vi "backemfconstant.vi"(4 "Cutoff Frequency":i32=10000, 6 "Noise Band":dbl=0.01, 7 "rate":i32=100000, 8 "Pole Pair":i32=5, 9 "Back  EMF data":dbl[](array[numeric])) -> (0 "Variance":dbl=3.1792063558717476e-05, 1 "ZCP":i32[](array[numeric]), 2 "Filiter Voltage":dbl[](array[numeric]), 3 "Mean":dbl=0.07460512010090932, 5 "B-EMF":dbl[](graph)=[0.07481589133166745, 0.07511337105786742, 0.0741529055838003, 0.07537265906376046, 0.07508825632115766, 0.07557435638030187, 0.0743975577603694, 0.07492228255252237, 0.07463056189525759, 0.0758438201846894, 0.07482290613743812, 0.07511679185821236, 0.07415273237871953, 0.07537876454285714, 0.07509791250440986, 0.07558596112071256, 0.0743927080181082, 0.07491881845090724, 0.07463770660483883, 0.07585304335523971, 0.07481316335164553, 0.07513961162760209, 0.07414004510655407, 0.0753934869747215, 0.07509271635198714, 0.07559592041285612, 0.07439296782572931, 0.07493276145990817, 0.07463588795149087, 0.07587720546400528, 0.07480203492520691, 0.07514974412482635, 0.07413324680713437, 0.07542358135750299, 0.07508440250811083, 0.07560570649991886, 0.07438603962249907, 0.07495536472294693, 0.07461891385357669, 0.07588144898848384, 0.07480381027728465, 0.07516195508301972, 0.07413138485251623, 0.07541942443556485, 0.07507565565153261, 0.07562294040545418, 0.07437421837573739, 0.07496484770111837, 0.07462229135265147, 0.07589993863085463, 0.07480216482901747, 0.07518568417908342, 0.07412164206672368, 0.07543691814872129, 0.07506110642474902, 0.07564398482276614, 0.07437668654813819, 0.07498160529268162, 0.07461267847066942, 0.0759097247179174, 0.07477362929196277, 0.07519404132422994, 0.07411445405587225, 0.07546108025748688, 0.07506634587844192, 0.07565281828188475, 0.07436131459722098, 0.07499658753216708, 0.07460471103695462, 0.07593150525682257, 0.0747739324008541, 0.07521118862722488, 0.07411661911938174, 0.075469350800093, 0.07505032440847191, 0.07567741340335221, 0.07435451629780128, 0.07502092284601342, 0.07459782613499454, 0.0759478731369541, 0.07476483913411439, 0.07523058759626963, 0.07409336633729012, 0.07548000291255955, 0.07504733662082885, 0.07569139971362333, 0.07435061918348428, 0.0750335235156385, 0.0745818912675649, 0.07596948047077853, 0.07476141833376944, 0.07525267124406612, 0.07408821348613759, 0.07550827864199311, 0.07503378332325962, 0.07571058217631717, 0.07433632976432183, 0.07505898466250974, 0.0745710659500176, 0.07598351008231984, 0.07475838724485617, 0.07526722047084973, 0.07407912021939786, 0.07552399700307182, 0.07501602980248206, 0.07573383495840878, 0.0743232094794545, 0.07508344988016666, 0.07455508778131775, 0.07600464110217219, 0.07473353231576757, 0.07529501988631122, 0.07406253583291537, 0.0755460806508683, 0.07500832217638835, 0.07575197819061805, 0.07430298778627613, 0.07510068378570196, 0.0745526629101872, 0.07604226990596659, 0.0747173376407168, 0.07531303321470993, 0.07405010836837107, 0.07557439968157206, 0.074991304777204, 0.07578306850261392, 0.07429489044875075, 0.0751250624008185, 0.07452858740396197, 0.07605456746670036, 0.07470581950284645, 0.0753423914758982, 0.07402646587484775, 0.07559358214426588, 0.07497147279545732, 0.07580671099613724, 0.07426800035996324, 0.07516173857666877, 0.07450693676886735, 0.07607426954463645, 0.07468577101474887, 0.07537097031422309, 0.07399957578606026, 0.07563593078651094, 0.07496328885539158, 0.0758321721430085, 0.07424877459599921, 0.07519157315182916, 0.07447896414832511, 0.07611419331575092, 0.07466234502757649, 0.07539301066074941, 0.07397181967186896, 0.07566411991340413, 0.07492154643092916, 0.07586607703756665, 0.0742194596360811, 0.07522162423334047, 0.07445055851508102, 0.07615680176561711, 0.07463056189525759, 0.07543172199629856, 0.07394415016021806, 0.07570560253024541, 0.0748928376887937, 0.07590998452553853, 0.07418278346023084, 0.07526743697720066, 0.07441184717953182, 0.07620157527899274, 0.07459211036732954, 0.0754861949941966, 0.07390513571577755, 0.075761114758628, 0.07485213449481584, 0.07596172954341465, 0.07414134414465974, 0.07530259760859431, 0.0])   [LabVIEW 2013]
uses:
  <vilib>/Analysis/NI_AALBase.lvlib
panel:
  out "standard deviation":dbl format="%0.5f"
  out "B-EMF 2":dbl[](graph)=[0.07481589133166745, 0.07511337105786742, 0.0741529055838003, 0.07537265906376046, 0.07508825632115766, 0.07557435638030187, 0.0743975577603694, 0.07492228255252237, 0.07463056189525759, 0.0758438201846894, 0.07482290613743812, 0.07511679185821236, 0.07415273237871953, 0.07537876454285714, 0.07509791250440986, 0.07558596112071256, 0.0743927080181082, 0.07491881845090724, 0.07463770660483883, 0.07585304335523971, 0.07481316335164553, 0.07513961162760209, 0.07414004510655407, 0.0753934869747215, 0.07509271635198714, 0.07559592041285612, 0.07439296782572931, 0.07493276145990817, 0.07463588795149087, 0.07587720546400528, 0.07480203492520691, 0.07514974412482635, 0.07413324680713437, 0.07542358135750299, 0.07508440250811083, 0.07560570649991886, 0.07438603962249907, 0.07495536472294693, 0.07461891385357669, 0.07588144898848384, 0.07480381027728465, 0.07516195508301972, 0.07413138485251623, 0.07541942443556485, 0.07507565565153261, 0.07562294040545418, 0.07437421837573739, 0.07496484770111837, 0.07462229135265147, 0.07589993863085463, 0.07480216482901747, 0.07518568417908342, 0.07412164206672368, 0.07543691814872129, 0.07506110642474902, 0.07564398482276614, 0.07437668654813819, 0.07498160529268162, 0.07461267847066942, 0.0759097247179174, 0.07477362929196277, 0.07519404132422994, 0.07411445405587225, 0.07546108025748688, 0.07506634587844192, 0.07565281828188475, 0.07436131459722098, 0.07499658753216708, 0.07460471103695462, 0.07593150525682257, 0.0747739324008541, 0.07521118862722488, 0.07411661911938174, 0.075469350800093, 0.07505032440847191, 0.07567741340335221, 0.07435451629780128, 0.07502092284601342, 0.07459782613499454, 0.0759478731369541, 0.07476483913411439, 0.07523058759626963, 0.07409336633729012, 0.07548000291255955, 0.07504733662082885, 0.07569139971362333, 0.07435061918348428, 0.0750335235156385, 0.0745818912675649, 0.07596948047077853, 0.07476141833376944, 0.07525267124406612, 0.07408821348613759, 0.07550827864199311, 0.07503378332325962, 0.07571058217631717, 0.07433632976432183, 0.07505898466250974, 0.0745710659500176, 0.07598351008231984, 0.07475838724485617, 0.07526722047084973, 0.07407912021939786, 0.07552399700307182, 0.07501602980248206, 0.07573383495840878, 0.0743232094794545, 0.07508344988016666, 0.07455508778131775, 0.07600464110217219, 0.07473353231576757, 0.07529501988631122, 0.07406253583291537, 0.0755460806508683, 0.07500832217638835, 0.07575197819061805, 0.07430298778627613, 0.07510068378570196, 0.0745526629101872, 0.07604226990596659, 0.0747173376407168, 0.07531303321470993, 0.07405010836837107, 0.07557439968157206, 0.074991304777204, 0.07578306850261392, 0.07429489044875075, 0.0751250624008185, 0.07452858740396197, 0.07605456746670036, 0.07470581950284645, 0.0753423914758982, 0.07402646587484775, 0.07559358214426588, 0.07497147279545732, 0.07580671099613724, 0.07426800035996324, 0.07516173857666877, 0.07450693676886735, 0.07607426954463645, 0.07468577101474887, 0.07537097031422309, 0.07399957578606026, 0.07563593078651094, 0.07496328885539158, 0.0758321721430085, 0.07424877459599921, 0.07519157315182916, 0.07447896414832511, 0.07611419331575092, 0.07466234502757649, 0.07539301066074941, 0.07397181967186896, 0.07566411991340413, 0.07492154643092916, 0.07586607703756665, 0.0742194596360811, 0.07522162423334047, 0.07445055851508102, 0.07615680176561711, 0.07463056189525759, 0.07543172199629856, 0.07394415016021806, 0.07570560253024541, 0.0748928376887937, 0.07590998452553853, 0.07418278346023084, 0.07526743697720066, 0.07441184717953182, 0.07620157527899274, 0.07459211036732954, 0.0754861949941966, 0.07390513571577755, 0.075761114758628, 0.07485213449481584, 0.07596172954341465, 0.07414134414465974, 0.07530259760859431, 0.0]
  out "Waveform Graph 2":dbl[][](graph)
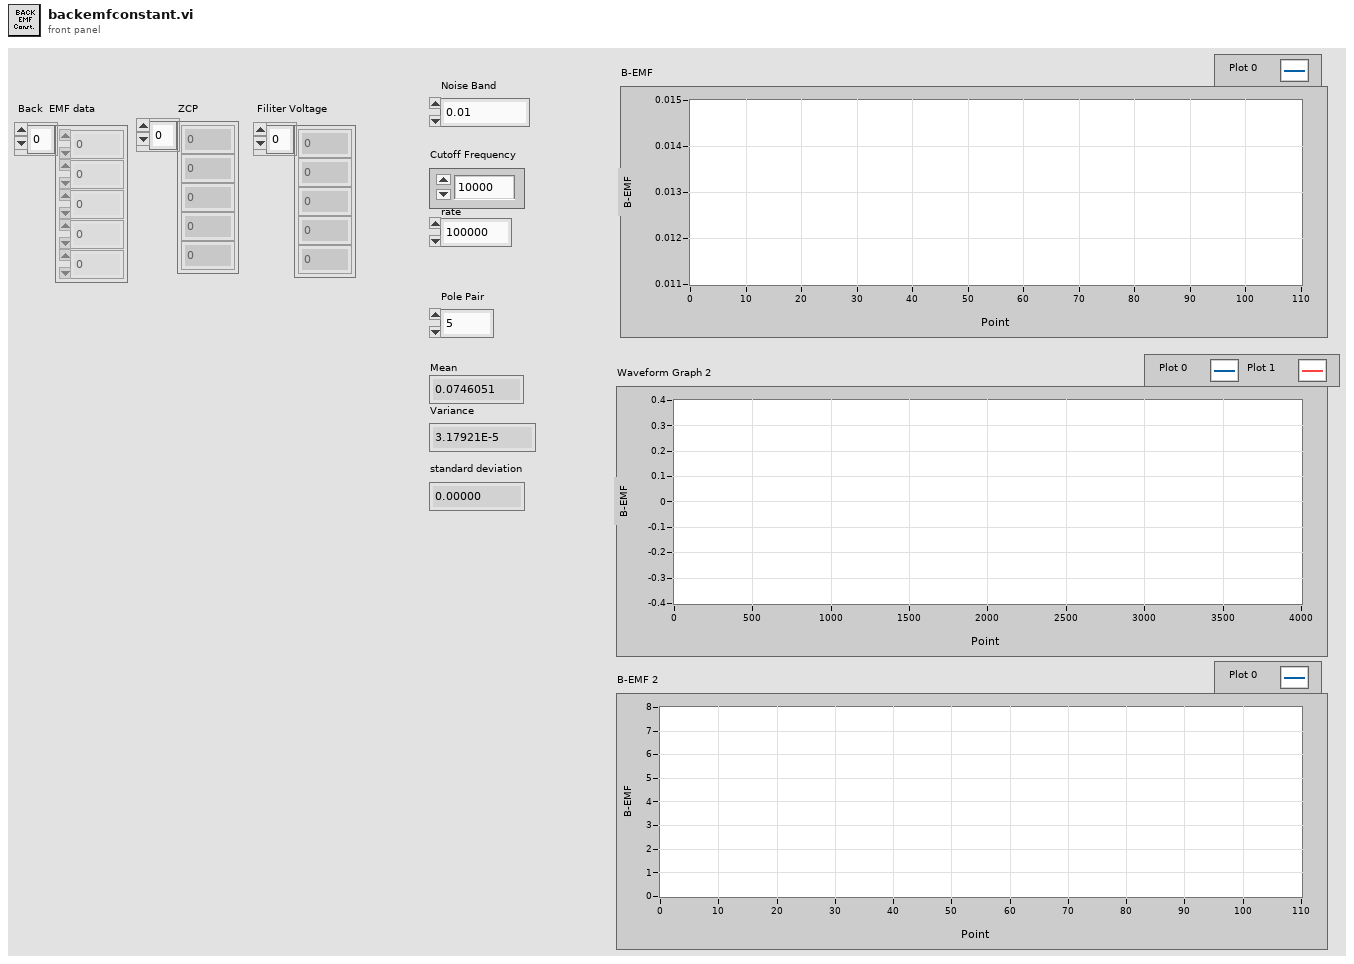
[diagram p1: front panel]
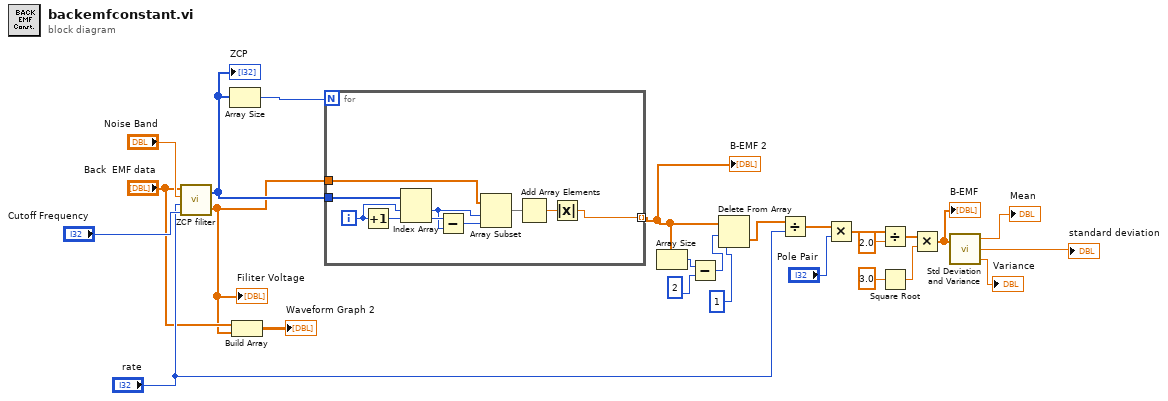
[diagram p0: block diagram]
diagram:
  n1 = call "ZCP filiter.vi"("Cutoff Frequency"="Cutoff Frequency", "Sampling Frequency"="rate", "Noise Band"="Noise Band", "Data"="Back  EMF data") -> ("Filiter Voltage"=w4:dbl[], "ZCP"=w24:i32[])
  "ZCP" <- w24
  "Filiter Voltage" <- w4
  n2 = Array Size(array=w24) -> (size(s)=w7:i32)
  n3 = Build Array("Back  EMF data", w4) -> (→"Waveform Graph 2":dbl[][])
  n4 = for {
    N: w7 -> [_]
    tunnel: w24 -> [w35]
    tunnel: w4 -> [w33]
    tunnel: [w26] -> w6 mode=indexing
    i -> [w34]
    n5 = Increment(x=w34) -> (x+1=w27:i32)
    n6 = Index Array(array=w35, index #1=w34, index #2=w27) -> (element #1=w31:i32, element #2=w32:i32)
    n7 = Subtract(x=w32, y=w31) -> (x-y=w30:i32)
    n8 = Array Subset(array=w33, index=w31, length=w30) -> (w29:dbl[])
    n9 = Add Array Elements(numeric array=w29) -> (sum=w28:dbl)
    n10 = Absolute Value(x=w28) -> (abs(x)=w26:dbl)
  }
  "B-EMF 2" <- w6
  n11 = Array Size(array=w6) -> (size(s)=w9:i32)
  n12 = Subtract(x=w9, y=2 ("length")) -> (x-y=w3:i32)
  n13 = Delete From Array(array=w6, length=w3, index=1 ("length")) -> (deleted portion=w1:dbl[])  [unwired: 1 out]
  n14 = Divide(x=w1, y="rate") -> (x/y=w23:dbl[])
  n15 = Multiply(x=w23, y="Pole Pair") -> (x*y=w22:dbl[])
  n16 = Divide(x=w22, y=2.0) -> (x/y=w18:dbl[])
  n17 = Square Root(x=3.0) -> (sqrt(x)=w20:dbl)
  n18 = Multiply(x=w18, y=w20) -> (x*y=w15:dbl[])
  "B-EMF" <- w15
  n19 = call <vilib>:"Std Deviation and Variance.vi"("X"=w15) -> ("mean"=→"Mean":dbl, "standard deviation"=→"standard deviation":dbl, "variance"=→"Variance":dbl)  [unwired: 1 in]
